vi "MS Operation IOP Ctrl_backup.vi"(6 "PID Cluster":T3={"L1 to L4 PID Cluster"={"L1 PID Gains"={"Kp"=0.005, "Kd"=0.5, "Ki"=0.0005}, "L2 PID Gains"={"Kp"=0.01, "Kd"=1.0, "Ki"=0.005}, "L3 PID Gains"={"Kp"=0.05, "Kd"=1.0, "Ki"=0.0005}, "L4 PID Gains"={"Kp"=0.1, "Kd"=0.1, "Ki"=0.0005}}, "Stage PID Cluster"={"Stage Z PID"={"Kp"=0.0005, "Kd"=0.001, "Ki"=0.0}, "Stage Y PID"={"Kp"=0.0003, "Kd"=0.01, "Ki"=0.0}, "Stage X PID"={"Kp"=0.0003, "Kd"=0.01, "Ki"=0.0}}, "OCT Z PID Gains"={"Kp"=0.0003, "Kd"=0.0001, "Ki"=0.01}}, 8 "error in":errorcluster, 9 "Offset Home 2 RCM":dbl[](array[numeric])=[0.0, 0.0, 0.0, 0.0], 10 "Prev Posit Cluster":T2={"Prev L1 to L4 Posit"=[-0.5319, -0.035669172703475985, -2.0566170657346783, 0.9099264705882353], "Prev Stage Posit"=[6.002553885707208, 5.996566124542428, 5.995469940427586], "Prev OCT Z Posit"=-0.0}, 11 "FPGA VI Reference In":refnum<k20>) -> (0 "error out":errorcluster, 2 "Last Posit Cluster":T1={"Last L1 to L4 Posit"=[0.0, 0.0, 0.0, 0.0], "Last Stage Posit"=[6.0, 6.0, 6.0], "Last OCT Z Posit"=0.0}, 3 "FPGA VI Reference Out":refnum<k20>)   [LabVIEW 2016]
uses:
  Global Variables.vi
  <vilib>/Platform/TimedLoop/XDataNode/wakeup.ctl
  <vilib>/Platform/TimedLoop/XDataNode/XDNodeRunTimeDep.lvlib
  <vilib>/Platform/TimedLoop/XDataNode/nitl_modes.ctl
  <vilib>/Platform/TimedLoop/XDataNode/timing_clust.ctl
  <vilib>/platform/TimedLoop/XDataNode/XDataNode.xnode
  <vilib>/rvi/interface/nirviReadWriteControl/nirviReadWriteControl.xnode
  Library/KevinLibraryAll/labview/KevLib01.lvlib
  FPGA Bitfiles/PhantomControlPI_FPGATarget_QuadCtr2_E2412E44.lvbitx
  IRISS_FPGA_IO.vi
  <vilib>/Utility/error.llb/Error Cluster From Error Code.vi
  <vilib>/rvi/errors/niLvFpgaAdjustHostInterfaceError.vi
  <vilib>/Utility/file.llb/Write Delimited Spreadsheet (DBL).vi
  <vilib>/Utility/file.llb/Write Delimited Spreadsheet (string).vi
  Library/KevinLibraryAll/labview2011/kevLib2011.lvlib
  NiFpgaLv.dll
panel:
  out "Period [ms]":i64=10
  out "Acc Ctrl Array":dbl[](array[numeric])
  out "Acc Button 4":bool
  out "Accurus Remote cmd":T4
  out "L1 to L4 Remote cmd":sgl[](array[numeric])
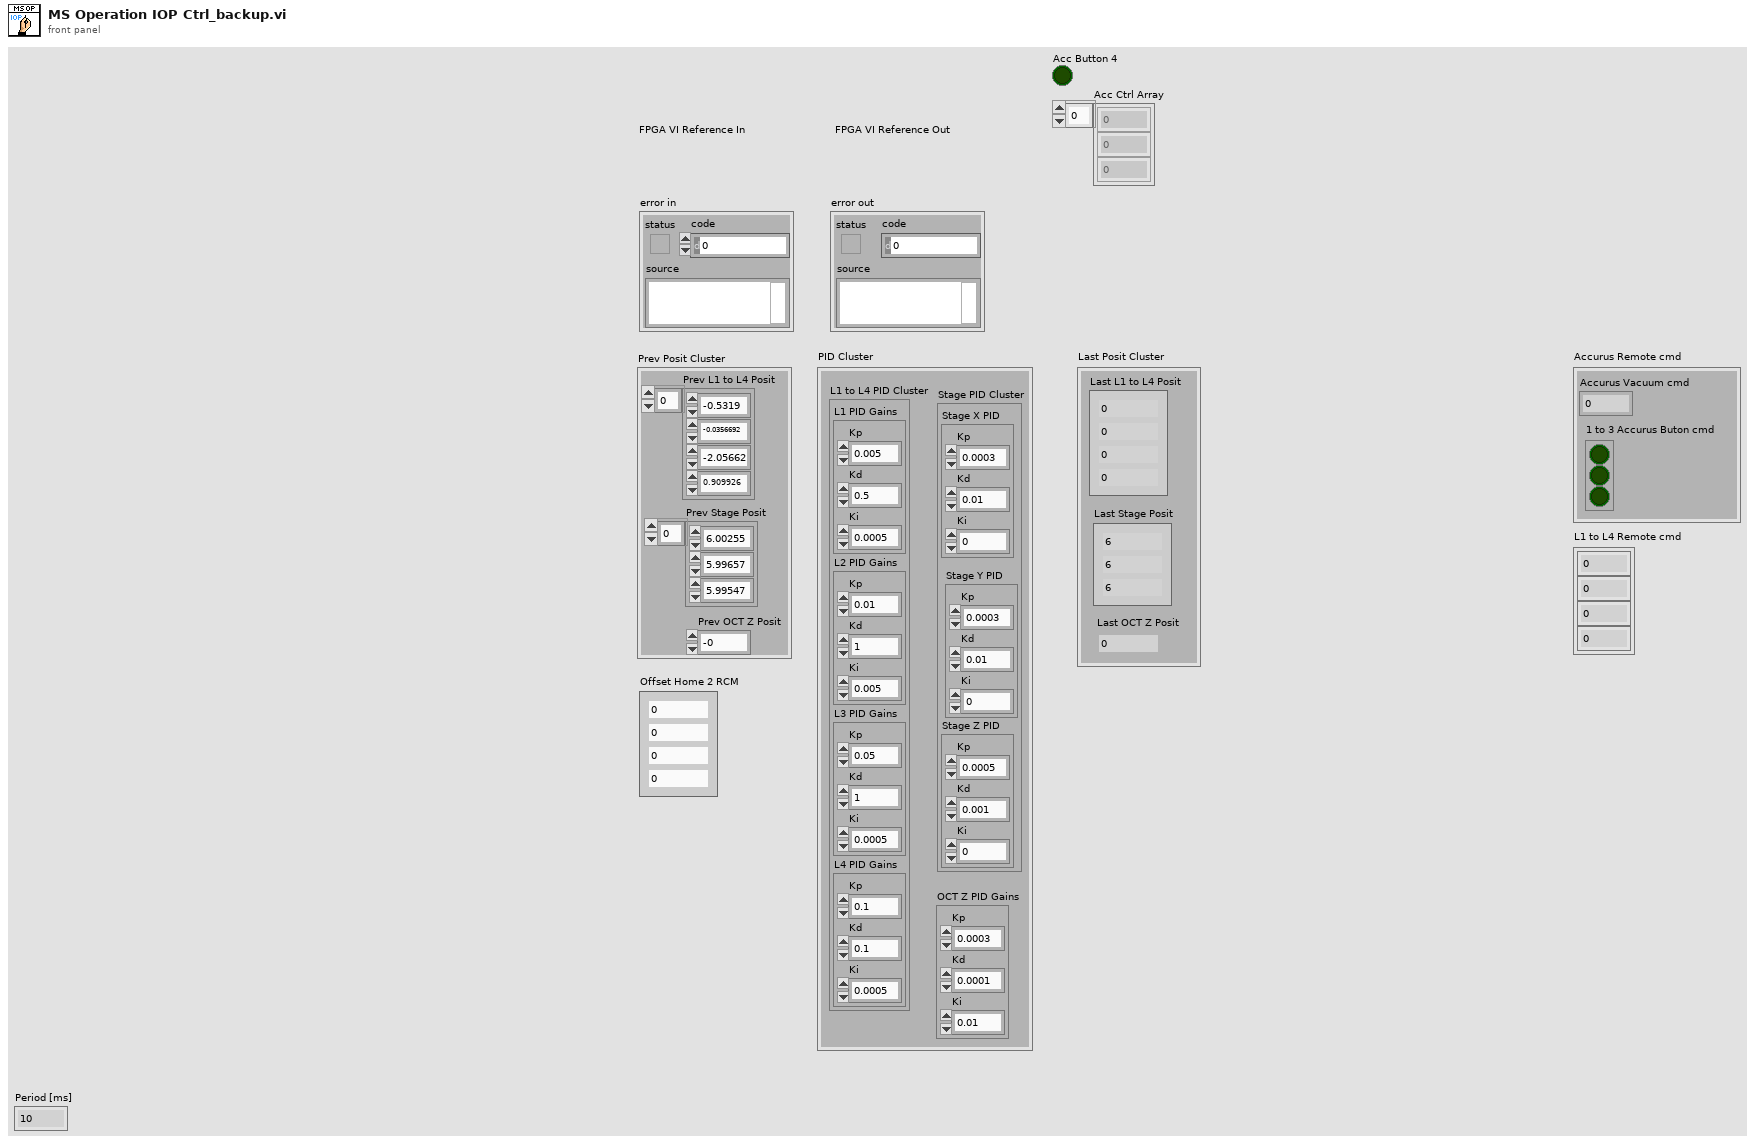
[diagram p1: front panel]
types:
  T1 = cluster{"Last L1 to L4 Posit":dbl[], "Last Stage Posit":dbl[], "Last OCT Z Posit":dbl}
  T2 = cluster{"Prev L1 to L4 Posit":dbl[], "Prev Stage Posit":dbl[], "Prev OCT Z Posit":dbl}
  T3 = cluster{"L1 to L4 PID Cluster":cluster{"L1 PID Gains":cluster{"Kp":dbl, "Kd":dbl, "Ki":dbl}, "L2 PID Gains":cluster{"Kp":dbl, "Kd":dbl, "Ki":dbl}, "L3 PID Gains":cluster{"Kp":dbl, "Kd":dbl, "Ki":dbl}, "L4 PID Gains":cluster{"Kp":dbl, "Kd":dbl, "Ki":dbl}}, "Stage PID Cluster":cluster{"Stage Z PID":cluster{"Kp":dbl, "Kd":dbl, "Ki":dbl}, "Stage Y PID":cluster{"Kp":dbl, "Kd":dbl, "Ki":dbl}, "Stage X PID":cluster{"Kp":dbl, "Kd":dbl, "Ki":dbl}}, "OCT Z PID Gains":cluster{"Kp":dbl, "Kd":dbl, "Ki":dbl}}
  T4 = cluster{"Accurus Vacuum cmd":sgl, "1 to 3 Accurus Buton cmd":bool[]}
  T5 = cluster{"Accurus button":bool[], "Accurus engaged?":bool, "Vacuum Force":i32, "Accurus Ch. A Vout":dbl, "Accurus Ch. B Vout":dbl, "Irrigation engaged?":bool}
  T6 = typedef "XDNodeRunTimeDep.lvlib/timing_clust.ctl" = cluster{"Expected End [f-1]":u64, "Actual End [f-1]":u64, "Finished Late? [f-1]":bool, "Expected End [i-1]":u64, "Actual End [i-1]":u64, "Finished Late? [i-1]":bool, "Expected Start [i]":u64, "Actual Start [i]":u64, "Expected Start [f]":u64, "Actual Start [f]":u64, "Source Name":string, "Structure Name":string, "Period":i64, "Deadline":i64, "Offset":i64, "Start":i64, "Priority":i32, "Timeout":i32, "Mode":T7, "Wakeup Reason":T8, "Error":errorcluster, "Source Type":string, "Secondary Source Type":string, "Global End Time":u64, "Global Start Time":u64, "Frame Duration":u64, "Iteration Duration":u64, "Assigned CPU":i32, "I/O Scan Engine Mode":u32}
  T7 = typedef "XDNodeRunTimeDep.lvlib/nitl_modes.ctl" = enum32{"No Change", "Process missed periods, maintain original phase", "Discard missed periods, maintain original phase", "Process missed periods, ignore original phase", "Discard missed periods, ignore original phase"}
  T8 = typedef "XDNodeRunTimeDep.lvlib/wakeup.ctl" = enum32{"Normal", "Aborted", "Asynchronous wakeup", "Timing source error", "Timed loop error", "Timeout"}
  T9 = cluster{"L1 PID Gains":cluster{"Kp":dbl, "Kd":dbl, "Ki":dbl}, "L2 PID Gains":cluster{"Kp":dbl, "Kd":dbl, "Ki":dbl}, "L3 PID Gains":cluster{"Kp":dbl, "Kd":dbl, "Ki":dbl}, "L4 PID Gains":cluster{"Kp":dbl, "Kd":dbl, "Ki":dbl}}
  T10 = cluster{"Stage Z PID":cluster{"Kp":dbl, "Kd":dbl, "Ki":dbl}, "Stage Y PID":cluster{"Kp":dbl, "Kd":dbl, "Ki":dbl}, "Stage X PID":cluster{"Kp":dbl, "Kd":dbl, "Ki":dbl}}
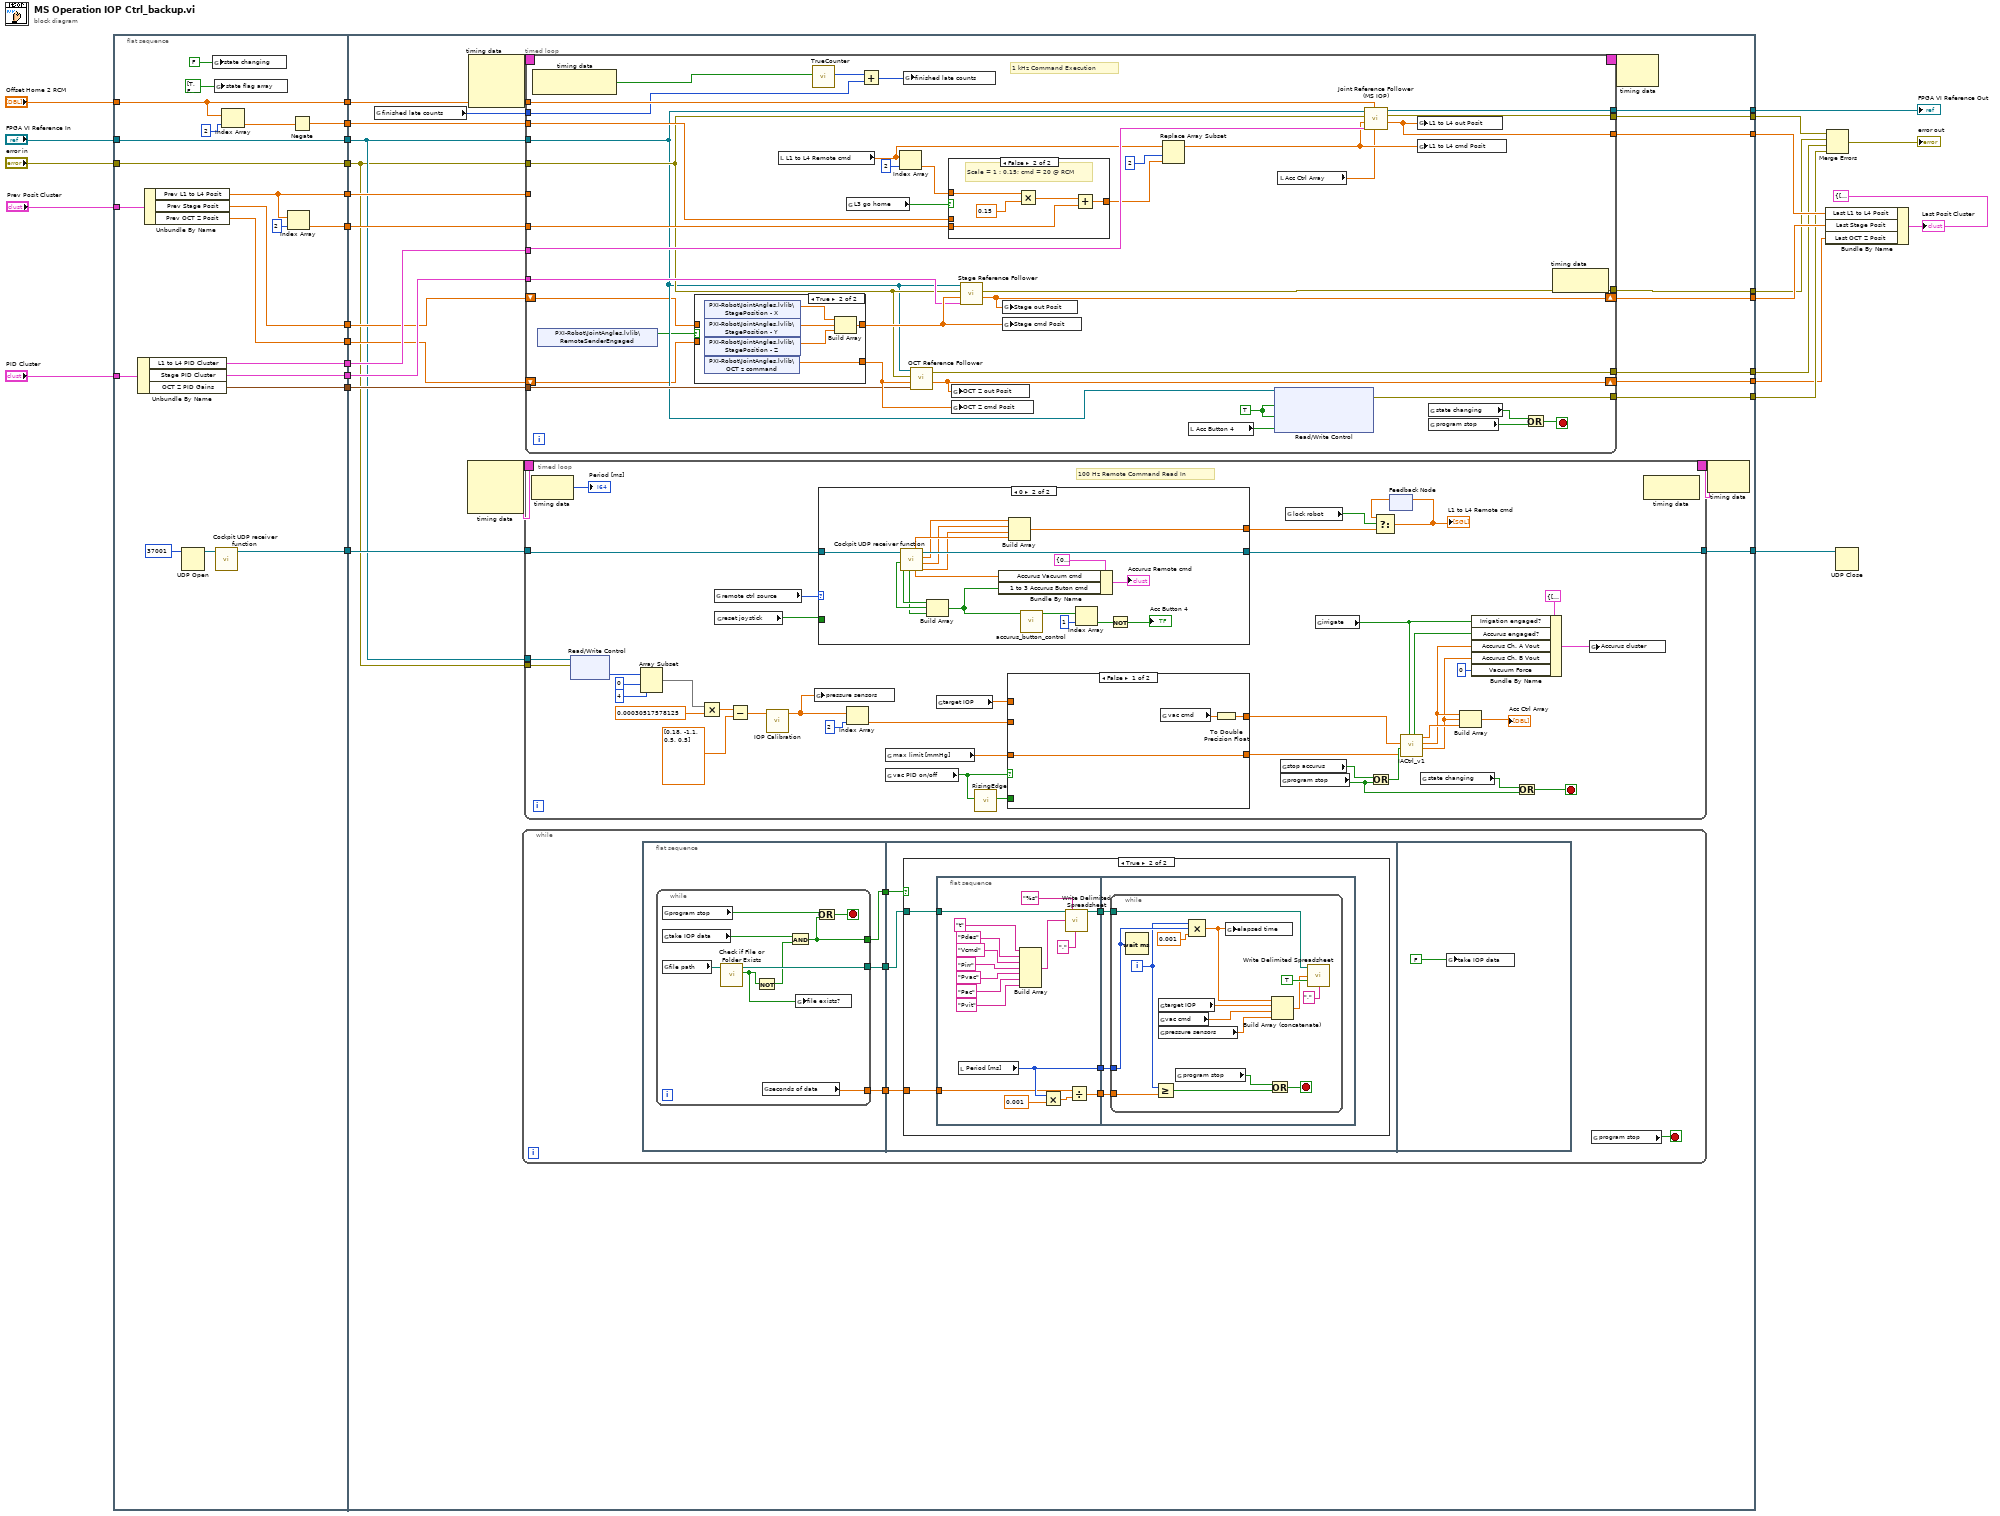
[diagram p0: block diagram]
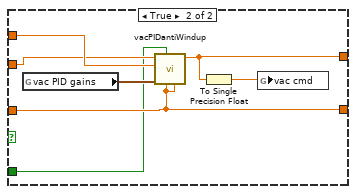
[diagram p3: hidden frame]
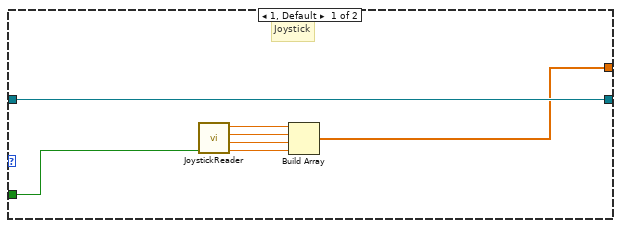
[diagram p4: hidden frame]
diagram:
  n1 = flat-sequence {
    tunnel: [w46] -> w29
    tunnel: [w45] -> w27
    tunnel: "FPGA VI Reference In" -> [w45]
    tunnel: [w44] -> w25
    tunnel: "error in" -> [w44]
    tunnel: [w37] -> w23
    tunnel: "Offset Home 2 RCM" -> [w37]
    tunnel: "Prev Posit Cluster" -> [w32]
    tunnel: [w42] -> w20
    tunnel: "PID Cluster" -> [w41]
    tunnel: [w40] -> w18
    tunnel: [w39] -> w17
    tunnel: [w35] -> w16
    tunnel: [w34] -> w4
    tunnel: [w33] -> w3
    tunnel: [w31] -> w2
    tunnel: [w30] -> w1
    tunnel: w29 -> [w72]
    tunnel: [w71] -> w28
    tunnel: w27 -> [w52]
    tunnel: w25 -> [w51]
    tunnel: w23 -> [w70]
    tunnel: w20 -> [w69]
    tunnel: w18 -> [w68]
    tunnel: w17 -> [w67]
    tunnel: w16 -> [w66]
    tunnel: [w65] -> w6
    tunnel: [w64] -> w12
    tunnel: [w63] -> w13
    tunnel: [w53] -> w10
    tunnel: [w54] -> w9
    tunnel: [w62] -> w7
    tunnel: [w61] -> w8
    tunnel: [w55] -> w5
    tunnel: w4 -> [w60]
    tunnel: w3 -> [w59]
    tunnel: w2 -> [w57]
    tunnel: w1 -> [w56]
    frame #0 {
      n2 = Unbundle By Name(w41) -> ("L1 to L4 PID Cluster"=w40:T9, "Stage PID Cluster"=w34:T10, "OCT Z PID Gains"=w33:cluster{"Kp":dbl, "Kd":dbl, "Ki":dbl})
      n3 = Unbundle By Name(w32) -> ("Prev L1 to L4 Posit"=w42:dbl[], "Prev Stage Posit"=w31:dbl[], "Prev OCT Z Posit"=w30:dbl)
      n4 = UDP Open(11:u16 37001 ("port")) -> (port=w48:refnum<k16>)  [unwired: 4 in, 2 out]
      n5 = global write "Global Variables.vi" "state changing"(FALSE ("state changing")) -> ()
      n6 = global write "Global Variables.vi" "state flag array"(bool[] [TRUE, FALSE, FALSE, FALSE, FALSE, FALSE, FALSE, FALSE, FALSE] ("state flag array")) -> ()
      n7 = call "Cockpit UDP receiver function.vi"("UDP connection ID"=w48) -> ("UDP connection ID out"=w46:refnum<k16>)  [unwired: 1 in, 9 out]
      n8 = Index Array(array=w37, index=2) -> (element=w36:dbl)
      n9 = Index Array(array=w42, index=2) -> (element=w39:dbl)
      n10 = Negate(x=w36) -> (-x=w35:dbl)
    }
    frame #1 {
      n11 = global read "Global Variables.vi" "finished late counts"() -> (w58:u16)
      n12 = node-c288() -> (w74:T6)  [unwired: 3 in]
      n13 = node-c288() -> (w76:T6)  [unwired: 3 in]
      n14 = while {
        stop <- w77 stop-if-true
        n15 = flat-sequence {
          tunnel: [w81] -> w80
          tunnel: [w83] -> w79
          tunnel: [w82] -> w78
          tunnel: w80 -> [w95]
          tunnel: w79 -> [w94]
          tunnel: w78 -> [w93]
          frame #0 {
            n16 = while {
              tunnel: [w91] -> w83
              tunnel: [w84] -> w82
              tunnel: [w89] -> w81
              stop <- w92 stop-if-true
              n17 = global read "Global Variables.vi" "program stop"() -> (w88:bool)
              n18 = global read "Global Variables.vi" "take IOP data"() -> (w87:bool)
              n19 = global read "Global Variables.vi" "file path"() -> (w86:path)
              n20 = call <vilib>:"Check if File or Folder Exists.vi"("path"=w86) -> ("file or folder exists?"=w85:bool, "dup path"=w91:path)  [unwired: 8 in, 1 out]
              n21 = Not(x=w85) -> (.not. x?=w90:bool)
              n22 = global read "Global Variables.vi" "seconds of data"() -> (w84:sgl)
              n23 = And(x=w87, y=w90) -> (x .and. y?=w89:bool)
              n24 = global write "Global Variables.vi" "file exists?"(w85) -> ()
              n25 = Or(x=w88, y=w89) -> (x .or. y?=w92:bool)
            }
          }
          frame #1 {
            n26 = case shown="True" w95 {
              tunnel: w94 -> [_ w100]
              tunnel: w93 -> [_ w97]
              frame False {
              }
              frame True {
                n27 = flat-sequence {
                  tunnel: w100 -> [w106]
                  tunnel: [w104] -> w99
                  tunnel: [w115] -> w98
                  tunnel: w97 -> [w114]
                  tunnel: [w112] -> w96
                  tunnel: w99 -> [w120]
                  tunnel: w98 -> [w119]
                  tunnel: w96 -> [w118]
                  frame #0 {
                    n28 = local read "Period [ms]"() -> (w115:i64)
                    n29 = Build Array("t" ("delimiter (\\t)"), "Pdes" ("delimiter (\\t)"), "Vcmd" ("delimiter (\\t)"), "Pirr" ("delimiter (\\t)"), "Pvac" ("delimiter (\\t)"), "Pac" ("delimiter (\\t)"), "Pvit" ("delimiter (\\t)")) -> (w103:string[])
                    n30 = Multiply(x=w115, y=0.001) -> (x*y=w113:dbl)
                    n31 = call-poly <vilib>:"Write Delimited Spreadsheet.vi"("file path (dialog if empty)"=w106, "format (%s)"="%s", "1D data"=w103, "delimiter (\\t)"="," ("delimiter (\\t)")) -> ("new file path (Not A Path if cancelled)"=w104:path)  [unwired: 10 in, 1 out]
                    n32 = Divide(x=w114, y=w113) -> (x/y=w112:dbl)
                  }
                  frame #1 {
                    n33 = while {
                      tunnel: w120 -> [w129]
                      tunnel: w119 -> [w133]
                      tunnel: w118 -> [w131]
                      i -> [w132]
                      stop <- w135 stop-if-true
                      n34 = Wait (ms)(milliseconds to wait=w133) -> ()  [unwired: 1 out]
                      n35 = Greater Or Equal?(x=w132, y=w131) -> (x >= y?=w130:bool)
                      n36 = global read "Global Variables.vi" "target IOP"() -> (w121:sgl)
                      n37 = global read "Global Variables.vi" "vac cmd"() -> (w124:sgl)
                      n38 = global read "Global Variables.vi" "pressure sensors"() -> (w123:sgl[])
                      n39 = global read "Global Variables.vi" "program stop"() -> (w125:bool)
                      n40 = Compound Arithmetic op=MULTIPLY(w132, w133, 0.001 ("y")) -> (w122:dbl)
                      n41 = global write "Global Variables.vi" "elapsed time"(w122) -> ()
                      n42 = Or(x=w125, y=w130) -> (x .or. y?=w135:bool)
                      n43 = Build Array (concatenate)(w122, w121, w124, w123) -> (w127:dbl[])
                      n44 = call-poly <vilib>:"Write Delimited Spreadsheet.vi"("file path (dialog if empty)"=w129, "1D data"=w127, "append to file? (new file:F)"=TRUE, "delimiter (\\t)"="," ("delimiter (\\t)")) -> ()  [unwired: 10 in, 2 out]
                    }
                  }
                }
              }
            }
          }
          frame #2 {
            n45 = global write "Global Variables.vi" "take IOP data"(FALSE) -> ()
          }
        }
        n46 = global read "Global Variables.vi" "program stop"() -> (w77:bool)
      }
      n47 = timed-loop {
        timing: w74 -> [_]
        timing-out: [_] -> w73
        tunnel: w72 -> [w176]
        tunnel: [w175] -> w71
        tunnel: w52 -> [w167]
        tunnel: w51 -> [w166]
        stop <- w178 stop-if-true
        # "100 Hz Remote Command Read In"
        n48 = node-c288() -> (→"Period [ms]":i64)  [unwired: 1 in]
        n49 = xnode "Read/Write Control"("FPGA VI Reference In"=w167, "error in"=w166) -> ("AI"=w158:i16[])  [unwired: 2 out]
        n50 = Array Subset(array=w158, index=0, length=4) -> (w163:i16[])
        n51 = Multiply(x=w163, y=0.00030517578125) -> (x*y=w164:dbl[])
        n52 = global read "Global Variables.vi" "remote ctrl source"() -> (w174:u16)
        n53 = global read "Global Variables.vi" "reset joystick"() -> (w173:bool)
        n54 = Subtract(x=w164, y=dbl[] [0.18, -1.1, 0.5, 0.5]) -> (x-y=w159:dbl[])
        n55 = call "IOP Calibration.vi"("IOP Input [V]"=w159) -> ("IOP Output [mmHg]"=w148:dbl[])  [unwired: 10 in]
        n56 = global write "Global Variables.vi" "pressure sensors"(w148) -> ()
        n57 = case shown="0" w174 {
          tunnel: [w194 w213] -> w175
          tunnel: w176 -> [w194 w203]
          tunnel: w173 -> [w195 _]
          tunnel: [w189 w202] -> w169
          frame 1, Default {
            # "Joystick"
            n58 = call "JoystickReader.vi"("Reset"=w195) -> ("L4 [deg]"=w190:sgl, "L3 [0~100]"=w191:sgl, "L2 [deg]"=w192:sgl, "L1 [deg]"=w193:sgl)  [unwired: 7 in]
            n59 = Build Array(w193, w192, w191, w190) -> (w189:sgl[])
          }
          frame 0 {
            n60 = call "Cockpit UDP receiver function.vi"("UDP connection ID"=w203) -> ("L3"=w210:sgl, "L2"=w209:sgl, "L1"=w211:sgl, "UDP connection ID out"=w213:refnum<k16>, "down_pedal"=w201:sgl, "L4"=w212:sgl, "right_pedal"=w204:bool, "left_pedal"=w206:bool, "up_pedal"=w205:bool)  [unwired: 1 in, 1 out]
            n61 = Build Array(w206, w205, w204) -> (w196:bool[])
            n62 = Bundle By Name(cluster=T4 {"Accurus Vacuum cmd"=0.0, "1 to 3 Accurus Buton cmd"=[FALSE, FALSE, FALSE]} ("Accurus Cockpit cmd 2"), "Accurus Vacuum cmd"=w201, "1 to 3 Accurus Buton cmd"=w196) -> (→"Accurus Remote cmd":T4)
            n63 = Build Array(w211, w209, w210, w212) -> (w202:sgl[])
            n64 = call "accurus_button_control.vi"("Array in"=w196) -> ("Array out"=w199:bool[])  [unwired: 10 in]
            n65 = Index Array(array=w199, index=1) -> (element=w198:bool)
            n66 = Not(x=w198) -> (.not. x?=→"Acc Button 4":bool)
          }
        }
        n67 = Index Array(array=w148, index=2) -> (element=w156:dbl)
        n68 = global read "Global Variables.vi" "max limit [mmHg]"() -> (w150:dbl)
        n69 = global read "Global Variables.vi" "vac PID on/off"() -> (w139:bool)
        n70 = global read "Global Variables.vi" "target IOP"() -> (w155:sgl)
        n71 = call "RisingEdge.vi"("Signal In"=w139) -> ("Rising Edge"=w138:bool)  [unwired: 10 in]
        n72 = case shown="False" w139 {
          tunnel: w156 -> [_ w184]
          tunnel: w155 -> [_ w185]
          tunnel: [w179 w187] -> w137
          tunnel: w150 -> [w181 w183]
          tunnel: [w181 w183] -> w149
          tunnel: w138 -> [_ w182]
          frame False {
            n73 = global read "Global Variables.vi" "vac cmd"() -> (w180:sgl)
            n74 = To Double Precision Float(number=w180) -> (double precision float=w179:dbl)
          }
          frame True {
            n75 = global read "Global Variables.vi" "vac PID gains"() -> (w186:cluster{"Kp":dbl, "Kd":dbl, "Ki":dbl, "Ts":dbl})
            n76 = call "vacPIDantiWindup.vi"("Saturation U"=w183, "Saturation M"=w183, "Reset"=w182, "PID Gains"=w186, "Feedback"=w185, "Reference"=w184) -> ("Control"=w187:dbl)  [unwired: 5 in]
            n77 = To Single Precision Float(number=w187) -> (single precision float=w188:sgl)
            n78 = global write "Global Variables.vi" "vac cmd"(w188) -> ()
          }
        }
        n79 = global read "Global Variables.vi" "stop accurus"() -> (w168:bool)
        n80 = global read "Global Variables.vi" "program stop"() -> (w151:bool)
        n81 = global read "Global Variables.vi" "lock robot"() -> (w172:bool)
        n82 = global read "Global Variables.vi" "irrigate"() -> (w144:bool)
        n83 = Or(x=w168, y=w151) -> (x .or. y?=w152:bool)
        n84 = feedback #1() -> (w171:sgl[])  [unwired: 1 in]
        n85 = Select(t=w171, s=w172, f=w169) -> (s? t:f=w170:sgl[])
        "L1 to L4 Remote cmd" <- w170
        n86 = feedback-in #1(w170) -> ()
        n87 = call "IACtrl_v1.vi"("Irrigate?"=w144, "Max Limit [mmHg]"=w149, "E-Stop Vacuum"=w152, "Vacuum Force [mmHg]"=w137) -> ("Accurus ChB Vout"=w142:dbl, "Accurus ChA Vout"=w143:dbl, "Accurus Engaged Vout"=w154:dbl, "Accurus Engaged"=w145:bool)  [unwired: 2 in, 2 out]
        n88 = global read "Global Variables.vi" "state changing"() -> (w177:bool)
        n89 = Build Array(w143, w142, w154) -> (→"Acc Ctrl Array":dbl[])
        n90 = Bundle By Name(cluster=T5 {"Accurus button"=[FALSE, FALSE, FALSE], "Accurus engaged?"=FALSE, "Vacuum Force"=0, "Accurus Ch. A Vout"=0.0, "Accurus Ch. B Vout"=0.0, "Irrigation engaged?"=FALSE} ("Accurus Output Cluster"), "Irrigation engaged?"=w144, "Accurus engaged?"=w145, "Accurus Ch. A Vout"=w143, "Accurus Ch. B Vout"=w142, "Vacuum Force"=0) -> (w146:T5)
        n91 = Or(x=w177, y=w151) -> (x .or. y?=w178:bool)
        n92 = global write "Global Variables.vi" "Accurus cluster"(w146) -> ()
        n93 = node-c288() -> ()  [unwired: 1 in, 1 out]
      }
      n94 = timed-loop {
        timing: w76 -> [_]
        timing-out: [_] -> w75
        tunnel: w52 -> [w229]
        tunnel: w51 -> [w230]
        tunnel: w70 -> [w251]
        tunnel: w69 -> [_]
        tunnel: w68 -> [w248]
        tunnel: w67 -> [w247]
        tunnel: w66 -> [w244]
        tunnel: [w243] -> w65
        tunnel: [w242] -> w64
        tunnel: [w241] -> w63
        tunnel: [w240] -> w62
        tunnel: [w239] -> w61
        tunnel: w60 -> [w236]
        tunnel: w59 -> [w235]
        tunnel: w58 -> [w231]
        shift-right: [w225] -> w54
        shift-left: w57 -> [w228]
        shift-right: [w226] -> w55
        shift-left: w56 -> [w227]
        tunnel: [w222] -> w53
        stop <- w256 stop-if-true
        w238 = TRUE ("Conn0/DIO15 Button 4")
        # "1 kHz Command Execution"
        n95 = node-c288() -> (w234:bool)  [unwired: 1 in]
        n96 = shared-variable "PXI-Robot\\JointAngles.lvlib\\RemoteSenderEngaged"() -> (w224:bool)  [unwired: 1 in, 1 out]
        n97 = case shown="True" w224 {
          tunnel: [w258 w263] -> w250
          tunnel: [w257 w259] -> w249
          tunnel: w228 -> [w258 _]
          tunnel: w227 -> [w257 _]
          frame False {
          }
          frame True {
            n98 = shared-variable "PXI-Robot\\JointAngles.lvlib\\StagePosition - X"() -> (w260:dbl)  [unwired: 1 in, 1 out]
            n99 = shared-variable "PXI-Robot\\JointAngles.lvlib\\StagePosition - Y"() -> (w261:dbl)  [unwired: 1 in, 1 out]
            n100 = shared-variable "PXI-Robot\\JointAngles.lvlib\\StagePosition - Z"() -> (w262:dbl)  [unwired: 1 in, 1 out]
            n101 = shared-variable "PXI-Robot\\JointAngles.lvlib\\OCT z command"() -> (w259:dbl)  [unwired: 1 in, 1 out]
            n102 = Build Array(w260, w261, w262) -> (w263:dbl[])
          }
        }
        n103 = local read "L1 to L4 Remote cmd"() -> (w223:sgl[])
        n104 = call "TrueCounter.vi"("True?"=w234) -> ("True Count"=w232:u16)  [unwired: 10 in]
        n105 = global read "Global Variables.vi" "L3 go home"() -> (w254:bool)
        n106 = Add(x=w232, y=w231) -> (x+y=w233:u16)
        n107 = Index Array(array=w223, index=2) -> (element=w252:sgl)
        n108 = global write "Global Variables.vi" "finished late counts"(w233) -> ()
        n109 = call "OCT Reference Follower.vi"("OCT Z PID Gains"=w235, "OCT  Z cmd Posit [mm]"=w249, "error in"=w230, "FPGA VI Reference In"=w229) -> ("OCT  Z out Posit [mm]"=w226:dbl, "error out"=w240:errorcluster)  [unwired: 5 in, 1 out]
        n110 = case shown="False" w254 {
          tunnel: [w264 w269] -> w245
          tunnel: w252 -> [_ w266]
          tunnel: w247 -> [_ w265]
          tunnel: w244 -> [w264 _]
          frame True {
            # "Go Home"
          }
          frame False {
            # "Scale = 1 : 0.15; cmd = 20 @ RCM"
            n111 = Multiply(x=w266, y=0.15) -> (x*y=w268:dbl)
            n112 = Add(x=w268, y=w265) -> (x+y=w269:dbl)
          }
        }
        n113 = global write "Global Variables.vi" "OCT Z out Posit"(w226) -> ()
        n114 = global write "Global Variables.vi" "OCT Z cmd Posit"(w249) -> ()
        n115 = call "Stage Reference Follower.vi"("Stage PID Cluster"=w236, "Stage cmd Posit [mm]"=w250, "error in"=w230, "FPGA VI Reference In"=w229) -> ("Stage out Posit [mm]"=w225:dbl[], "error out"=w239:errorcluster)  [unwired: 5 in, 1 out]
        n116 = global write "Global Variables.vi" "Stage out Posit"(w225) -> ()
        n117 = global write "Global Variables.vi" "Stage cmd Posit"(w250) -> ()
        n118 = Replace Array Subset(array=w223, new element=w245, index=2) -> (w221:sgl[])
        n119 = local read "Acc Button 4"() -> (w219:bool)
        n120 = xnode "Read/Write Control"("FPGA VI Reference In"=w229, "Conn0/DIO12 Button 1"=w238, "Conn0/DIO13 Button 2"=w238, "Conn0/DIO15 Button 4"=w219) -> ("error out"=w243:errorcluster)  [unwired: 1 in, 1 out]
        n121 = local read "Acc Ctrl Array"() -> (w220:dbl[])
        n122 = call "Joint Reference Follower (MS IOP).vi"("Acc Ctrl Array"=w220, "Offset Home2RCM [deg/mm]"=w251, "PID Ctrl Cluster"=w248, "Ref Array [deg/mm]"=w221, "error in"=w230, "FPGA VI Reference In"=w229) -> ("Output Posit Array [deg/mm]"=w222:dbl[], "error out"=w242:errorcluster, "FPGA VI Reference Out"=w241:refnum<k20>)  [unwired: 3 in]
        n123 = global write "Global Variables.vi" "L1 to L4 out Posit"(w222) -> ()
        n124 = global write "Global Variables.vi" "L1 to L4 cmd Posit"(w221) -> ()
        n125 = global read "Global Variables.vi" "state changing"() -> (w255:bool)
        n126 = global read "Global Variables.vi" "program stop"() -> (w237:bool)
        n127 = Or(x=w255, y=w237) -> (x .or. y?=w256:bool)
        n128 = node-c288() -> ()  [unwired: 1 in, 1 out]
      }
      n129 = node-c288(w75) -> ()  [unwired: 1 out]
      n130 = node-c288(w73) -> ()  [unwired: 1 out]
    }
  }
  n131 = Bundle By Name(cluster=T1 {"Last L1 to L4 Posit"=[-0.5607, -0.038216970753724266, -2.0806193533568895, 1.1787683823529411], "Last Stage Posit"=[6.002553885707208, 5.996566124542428, 5.995469940427586], "Last OCT Z Posit"=-0.0} ("Last Posit Cluster 2"), "Last L1 to L4 Posit"=w10, "Last Stage Posit"=w9, "Last OCT Z Posit"=w5) -> (→"Last Posit Cluster":T1)
  n132 = Merge Errors(w12, w8, w7, w6) -> (→"error out":errorcluster)
  n133 = UDP Close(connection ID=w28) -> ()  [unwired: 1 in, 2 out]
  "FPGA VI Reference Out" <- w13
